vi "SetPosition.vi"(8 "error in (no error)":errorcluster, 10 "Position":T1, 11 "Fruit in":refnum<class "Fruit.lvclass">) -> (0 "error out":errorcluster, 3 "Fruit out":refnum<class "Fruit.lvclass">)   [LabVIEW 2021, in "Fruit.lvclass"]
uses:
  Fruit.lvclass
  SnakeGame/Position.ctl
  Fruit.lvclass/Fruit.ctl
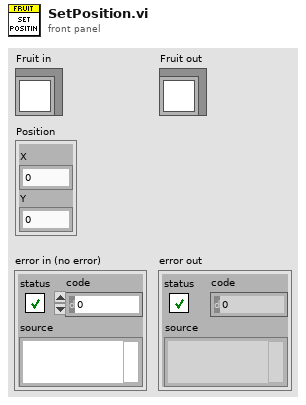
[diagram p1: front panel]
types:
  T1 = typedef "Position.ctl" = cluster{"X":i32, "Y":i32}
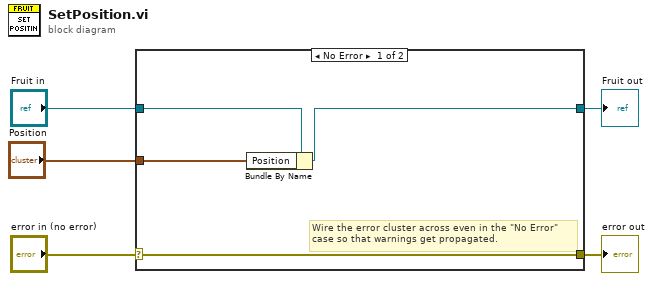
[diagram p0: block diagram]
diagram:
  n1 = case shown="No Error" "error in (no error)" {
    selector: "error in (no error)" -> [w9 w11]
    tunnel: [w9 w11] -> w4
    tunnel: [w8 w10] -> w2
    tunnel: "Fruit in" -> [w7 w10]
    tunnel: "Position" -> [w6 _]
    frame No Error {
      # "Wire the error cluster across even in the \"No Error\"\ncase so that warnings get propagated."
      n2 = Bundle By Name(cluster=w7, "Position"=w6) -> (w8:refnum<class "Fruit.lvclass">)
    }
    frame Error {
    }
  }
  "error out" <- w4
  "Fruit out" <- w2
